vi "Ignore nearby.vi"(2 "Pixel messurments":dbl[][](array[numeric])=[[23.153969547670897, -111.544571524119, 21.215260576456764, -113.32770834490657, 24.840963307768085, -109.79999757930636, 5.058701764442134, 2.0870321222371477], [23.050654694780935, -101.06514097376787, 21.607228439301235, -101.66666442528367, 24.351003479212505, -100.29477690532804, 3.0676337521043995, 16.638621652215505], [26.166824298370553, -72.64693767062666, 25.428915102034793, -73.44497830048203, 26.800802621990428, -71.87710684910417, 2.0833377679713307, 56.22134914640533], [29.98722136986337, -92.77263364027391, 29.544577661901695, -94.41525896266103, 30.426505353301746, -91.67148392274976, 2.8820301737661103, 93.58353525070883], [33.497201865026476, -86.57562011966348, 31.3084330447018, -87.45782939717174, 35.424095604568706, -85.39999811723828, 4.6014506281565986, 14.316750347188261], [33.5765445343372, -116.26011097886011, 31.896384838968494, -116.95341107621789, 35.4240956045687, -115.67951552197337, 3.750673689999642, 171.9805540666988], [38.33864305074378, -21.110133273436578, 37.0899590216577, -22.881123993545778, 39.931726027280085, -19.353413227945573, 4.529942931205161, 120.31992372552097], [40.0072805802987, -113.89413853927944, 38.9518063701689, -114.79758783057333, 40.81365371868012, -112.73975655063988, 2.775093714783486, 47.83521789725366], [41.038596937087156, -58.27234689395295, 40.42168585583566, -59.922087032347925, 41.891565341502414, -56.00240840390325, 4.186218610234045, 73.82475304681395], [45.0319078671391, -81.3913267852408, 44.04738858714698, -82.4602391459048, 46.00722790136932, -80.20642393454911, 2.9867462470905948, 50.627358900913684], [48.95238800468319, -102.12113110093198, 48.261043112725, -103.43051980808379, 49.534938666969516, -100.68674476817252, 3.0250803878184858, 94.7160819713975], [51.907561130887736, -82.82818937012169, 51.20080208405851, -83.93011863157155, 52.572689604014144, -81.8722873516381, 2.4732053986845846, 57.35545946274767], [58.16901076576446, -83.11221235775318, 57.27630395814775, -84.51807042583825, 59.04015934094785, -81.67630342021586, 3.3446712133895797, 115.97608069015298], [59.765299887202126, -69.69094378329712, 58.060239683836684, -72.26907471194865, 61.685942415148006, -67.46746839210392, 6.016738613784976, 59.86524109532162], [59.34002546551593, -97.34457616713128, 58.158231649547794, -99.70682511106135, 60.90200668945907, -95.2971866540611, 5.1935741826891935, 122.23317974279698], [61.1549553545596, -135.6886543755193, 58.746183443814495, -137.72770780697465, 63.939757626503685, -133.3180693499744, 6.8130847721536005, 15.222386784548284], [59.62811113521553, -72.96668418213245, 58.942167375236735, -73.83694616332652, 60.31405489519237, -72.36706667765976, 2.0106270339856613, 48.415236976347224], [62.824559752547245, -84.35320972876715, 62.07791027799247, -85.3999981172383, 63.93975762650369, -83.44015880301596, 2.703228752201658, 55.070701538642446], [67.50979258154165, -35.983900770382576, 66.19357283785939, -36.893975090235486, 68.83935591205955, -34.93413577601315, 3.2925883759278944, 28.854486763895764], [70.58563258349632, -102.94916232772741, 70.11325146630405, -103.92047963663937, 70.9951791577041, -102.05863228812815, 2.0601631008287864, 90.85123906790069], [72.09966487288538, -135.68357879336168, 70.70120326057074, -136.45381225273013, 73.444978300482, -134.98393276706338, 3.112691306895698, 158.10400496188345], [74.93335976567708, -53.65471277783657, 73.73895419761537, -54.72851284965874, 76.09076137468217, -52.180721741169705, 3.4673096963782624, 79.81300563717497], [81.4765115108334, -135.9072404854036, 80.89236769452688, -137.2377479784191, 82.06827128306028, -134.68995686993006, 2.806062861380964, 84.7022174765496], [86.0399891231283, -50.73731834562851, 84.71405435726045, -51.78875387832524, 87.55582136288284, -49.63293063268067, 3.566961393217694, 34.49100372630609], [86.52149180204897, -127.56713202513569, 85.49799008294937, -128.32047909870747, 87.65381332859394, -126.75260764732958, 2.665669663425548, 142.89159787285385], [87.31640917394765, -95.77322716932507, 86.37991777434944, -96.66907417401673, 88.14377315714954, -94.61124289408328, 2.7103238529934846, 57.3397049555742], [90.69523063175343, -49.389283942453375, 89.90762853994964, -50.80883422121407, 91.47549999132751, -48.0650591813028, 3.1601459393018283, 67.85295326199508], [91.47767759056437, -38.45930600916872, 90.59357229992747, -39.83373406156899, 92.25943571701644, -37.38393491879107, 2.9625355296351765, 67.4436053938025], [91.6756439590325, -110.08519117762921, 90.98554016277193, -111.46586099639536, 92.35742768272756, -108.82007792219521, 2.9803092864892458, 73.2743292894458], [94.97610203064093, -79.2583337845439, 93.92529913410543, -81.38232752308251, 96.08112237975, -77.2666649632156, 4.646100749354419, 82.72828659799865], [95.55597452715126, -53.02657057247167, 94.41525896266101, -53.84658515825869, 96.76706613972782, -52.27871370688082, 2.826520455639525, 27.994921080233407], [97.52458601055257, -59.89827657686741, 95.98313041403888, -61.48995848372581, 99.0208813510835, -58.06023968383672, 4.58158289260689, 67.83670357667657], [104.04356927261908, -97.09280280543281, 102.15662425383924, -99.31485724821688, 106.37027877941726, -95.2971866540611, 5.82207535712724, 139.97342300498846], [105.6341245242916, -56.8165471327239, 103.43051980808376, -59.62811113521459, 107.44819040223955, -54.14056105539205, 6.8010942414955915, 97.24255309011542], [108.74034645194116, -27.947236302017327, 107.15421450510621, -29.05461783334615, 110.09397347643971, -26.800802621990464, 3.7043036884783214, 179.48800650814684], [108.94516822485872, -101.74905431831091, 107.44819040223955, -103.03855194523932, 110.38794937357305, -100.29477690532805, 4.021254067971323, 134.86479080046723], [108.19190180442153, -38.31485859305124, 107.54618236795066, -40.4216858558357, 108.8200779221952, -36.40401526167991, 4.214793813019577, 95.766849041926], [113.34632336244485, -120.71810593844376, 108.33011809363958, -129.1044148243964, 119.99116201326248, -113.03373244777325, 19.855648499751403, 117.93513609604776], [110.89988870847331, -36.10088123691543, 110.19196544215083, -37.38393491879108, 111.95582082495093, -34.93413577601316, 3.01872516990009, 118.34762931907156], [112.12384659651235, -141.66925469877293, 110.1919654421508, -142.5293141268194, 113.81766817346212, -140.66746677830818, 4.075806158908521, 154.94585244328283], [111.94393422553061, -111.33684790541606, 111.17188509926198, -112.64176458492877, 112.93574048206209, -109.8979895450175, 3.261822693077137, 80.35839913755879], [113.17320881710795, -56.74212824263561, 112.05381279066204, -57.76626378670337, 114.50361193343996, -55.806424472481034, 3.1372736535927026, 35.50013253075657], [113.35459839606153, -104.14071410499425, 112.24979672208427, -105.39035912230612, 114.69959586486219, -103.23453587666155, 3.263294302758627, 143.00507300986496], [113.19783010478292, -99.25886183936566, 112.54377261921762, -100.0008010081947, 114.11164407059549, -98.53092152252795, 2.149131589835694, 47.55595083581141], [116.66657407075296, -129.615181166239, 114.69959586486218, -131.84818986430767, 118.9132503904402, -127.83051927015187, 5.8220753571272486, 34.29865811759245], [117.22479297101977, -102.7280748104678, 116.65943517908453, -104.21445553377274, 117.73734680190681, -100.78473673388365, 3.5951167592900255, 99.12601563426801], [117.88310678098033, -27.52604140581268, 116.85541911050677, -30.034537490457318, 119.01124235615134, -24.351003479212544, 6.078662083340181, 88.17913237932774], [120.27203997437059, -29.277282745526623, 119.59919415041804, -30.132529456168434, 121.0690736360848, -28.564658004790566, 2.149131589835694, 134.80702391388525], [122.37824080821565, -66.95925515815723, 120.77509773895143, -67.76144428923729, 123.81284867599605, -66.0955808721483, 3.4645391728065165, 2.419559816356106], [124.22781044838646, -130.0453519753959, 120.97108167037365, -133.41606131568554, 127.14457551017401, -126.94859157875183, 8.940927859467736, 49.997547132224106], [127.11854733497613, -75.26923831502631, 121.46104149892925, -85.79196598008278, 133.02409345284104, -64.9196772836149, 23.861194561831226, 100.51933634071696], [123.44513135008438, -88.742489220347, 121.55903346464036, -90.49558033421638, 125.08674423024057, -86.67389367148283, 5.200964544567394, 127.6966770746937], [123.85620676494109, -112.66471886731529, 122.83292901888488, -114.11164407059553, 124.79276833310722, -111.26987706497314, 3.452044300384267, 90.633155429399], [124.9514844539646, -25.088566629005186, 123.81284867599607, -26.89879458770158, 126.06666388735175, -23.371083822101376, 4.186218610234045, 93.52218227931537], [125.59434261258917, -97.05761231803307, 124.59678440168499, -98.04096169397238, 126.4586317501962, -96.17911434546116, 2.6330497713329524, 129.10781173086656], [127.40158171115596, -115.12378229825315, 126.06666388735174, -116.8554191105068, 128.9084308929741, -113.22971637919548, 4.606664738189911, 58.13558778744161], [128.23124963877498, -34.471450789306296, 127.24256747588515, -35.914055433124325, 129.10441482439637, -33.07228842750194, 3.397368873614151, 107.02312092204234], [129.10060076613485, -65.4422033045112, 128.32047909870744, -66.29156480357054, 129.8883505500853, -64.72369335219267, 2.2173050705961703, 39.82366841561815], [133.78792767072648, -31.77990687124756, 130.08433448150754, -35.13011970743539, 137.04176404699683, -29.15260979905727, 9.17259237421478, 123.5919624202362], [133.52789338380413, -130.03809978431872, 130.86827020719645, -133.2200773842633, 136.355820287019, -126.85059961304071, 8.407345178869432, 105.15474563599331], [133.4386543999588, -76.84519319023414, 132.24015772715208, -79.61847214028242, 134.4939729385078, -74.32690599188211, 5.75155242607024, 105.42860515334493], [136.10731294416433, -56.13063043246762, 133.71003721281886, -59.628111135214596, 138.80561942979693, -53.65060122683647, 7.854653578277136, 114.24744088018468], [138.67403021873304, -30.05693565405594, 138.11967566981912, -31.210441078990723, 139.1975872926414, -28.956625867635037, 2.498314726681498, 111.14098598849264]], 3 "Raw par mes.":dbl[][](array[numeric])=[[23.153969547670897, -111.544571524119, 21.215260576456764, -113.32770834490657, 24.840963307768085, -109.79999757930636, 5.058701764442134, 2.0870321222371477], [23.050654694780935, -101.06514097376787, 21.607228439301235, -101.66666442528367, 24.351003479212505, -100.29477690532804, 3.0676337521043995, 16.638621652215505], [26.166824298370553, -72.64693767062666, 25.428915102034793, -73.44497830048203, 26.800802621990428, -71.87710684910417, 2.0833377679713307, 56.22134914640533], [29.98722136986337, -92.77263364027391, 29.544577661901695, -94.41525896266103, 30.426505353301746, -91.67148392274976, 2.8820301737661103, 93.58353525070883], [33.497201865026476, -86.57562011966348, 31.3084330447018, -87.45782939717174, 35.424095604568706, -85.39999811723828, 4.6014506281565986, 14.316750347188261], [33.5765445343372, -116.26011097886011, 31.896384838968494, -116.95341107621789, 35.4240956045687, -115.67951552197337, 3.750673689999642, 171.9805540666988], [38.33864305074378, -21.110133273436578, 37.0899590216577, -22.881123993545778, 39.931726027280085, -19.353413227945573, 4.529942931205161, 120.31992372552097], [40.0072805802987, -113.89413853927944, 38.9518063701689, -114.79758783057333, 40.81365371868012, -112.73975655063988, 2.775093714783486, 47.83521789725366], [41.038596937087156, -58.27234689395295, 40.42168585583566, -59.922087032347925, 41.891565341502414, -56.00240840390325, 4.186218610234045, 73.82475304681395], [45.0319078671391, -81.3913267852408, 44.04738858714698, -82.4602391459048, 46.00722790136932, -80.20642393454911, 2.9867462470905948, 50.627358900913684], [48.95238800468319, -102.12113110093198, 48.261043112725, -103.43051980808379, 49.534938666969516, -100.68674476817252, 3.0250803878184858, 94.7160819713975], [51.907561130887736, -82.82818937012169, 51.20080208405851, -83.93011863157155, 52.572689604014144, -81.8722873516381, 2.4732053986845846, 57.35545946274767], [58.16901076576446, -83.11221235775318, 57.27630395814775, -84.51807042583825, 59.04015934094785, -81.67630342021586, 3.3446712133895797, 115.97608069015298], [59.765299887202126, -69.69094378329712, 58.060239683836684, -72.26907471194865, 61.685942415148006, -67.46746839210392, 6.016738613784976, 59.86524109532162], [59.34002546551593, -97.34457616713128, 58.158231649547794, -99.70682511106135, 60.90200668945907, -95.2971866540611, 5.1935741826891935, 122.23317974279698], [61.1549553545596, -135.6886543755193, 58.746183443814495, -137.72770780697465, 63.939757626503685, -133.3180693499744, 6.8130847721536005, 15.222386784548284], [59.62811113521553, -72.96668418213245, 58.942167375236735, -73.83694616332652, 60.31405489519237, -72.36706667765976, 2.0106270339856613, 48.415236976347224], [62.824559752547245, -84.35320972876715, 62.07791027799247, -85.3999981172383, 63.93975762650369, -83.44015880301596, 2.703228752201658, 55.070701538642446], [67.50979258154165, -35.983900770382576, 66.19357283785939, -36.893975090235486, 68.83935591205955, -34.93413577601315, 3.2925883759278944, 28.854486763895764], [70.58563258349632, -102.94916232772741, 70.11325146630405, -103.92047963663937, 70.9951791577041, -102.05863228812815, 2.0601631008287864, 90.85123906790069], [72.09966487288538, -135.68357879336168, 70.70120326057074, -136.45381225273013, 73.444978300482, -134.98393276706338, 3.112691306895698, 158.10400496188345], [74.93335976567708, -53.65471277783657, 73.73895419761537, -54.72851284965874, 76.09076137468217, -52.180721741169705, 3.4673096963782624, 79.81300563717497], [81.4765115108334, -135.9072404854036, 80.89236769452688, -137.2377479784191, 82.06827128306028, -134.68995686993006, 2.806062861380964, 84.7022174765496], [86.0399891231283, -50.73731834562851, 84.71405435726045, -51.78875387832524, 87.55582136288284, -49.63293063268067, 3.566961393217694, 34.49100372630609], [86.52149180204897, -127.56713202513569, 85.49799008294937, -128.32047909870747, 87.65381332859394, -126.75260764732958, 2.665669663425548, 142.89159787285385], [87.31640917394765, -95.77322716932507, 86.37991777434944, -96.66907417401673, 88.14377315714954, -94.61124289408328, 2.7103238529934846, 57.3397049555742], [90.69523063175343, -49.389283942453375, 89.90762853994964, -50.80883422121407, 91.47549999132751, -48.0650591813028, 3.1601459393018283, 67.85295326199508], [91.47767759056437, -38.45930600916872, 90.59357229992747, -39.83373406156899, 92.25943571701644, -37.38393491879107, 2.9625355296351765, 67.4436053938025], [91.6756439590325, -110.08519117762921, 90.98554016277193, -111.46586099639536, 92.35742768272756, -108.82007792219521, 2.9803092864892458, 73.2743292894458], [94.97610203064093, -79.2583337845439, 93.92529913410543, -81.38232752308251, 96.08112237975, -77.2666649632156, 4.646100749354419, 82.72828659799865], [95.55597452715126, -53.02657057247167, 94.41525896266101, -53.84658515825869, 96.76706613972782, -52.27871370688082, 2.826520455639525, 27.994921080233407], [97.52458601055257, -59.89827657686741, 95.98313041403888, -61.48995848372581, 99.0208813510835, -58.06023968383672, 4.58158289260689, 67.83670357667657], [104.04356927261908, -97.09280280543281, 102.15662425383924, -99.31485724821688, 106.37027877941726, -95.2971866540611, 5.82207535712724, 139.97342300498846], [105.6341245242916, -56.8165471327239, 103.43051980808376, -59.62811113521459, 107.44819040223955, -54.14056105539205, 6.8010942414955915, 97.24255309011542], [108.74034645194116, -27.947236302017327, 107.15421450510621, -29.05461783334615, 110.09397347643971, -26.800802621990464, 3.7043036884783214, 179.48800650814684], [108.94516822485872, -101.74905431831091, 107.44819040223955, -103.03855194523932, 110.38794937357305, -100.29477690532805, 4.021254067971323, 134.86479080046723], [108.19190180442153, -38.31485859305124, 107.54618236795066, -40.4216858558357, 108.8200779221952, -36.40401526167991, 4.214793813019577, 95.766849041926], [113.34632336244485, -120.71810593844376, 108.33011809363958, -129.1044148243964, 119.99116201326248, -113.03373244777325, 19.855648499751403, 117.93513609604776], [110.89988870847331, -36.10088123691543, 110.19196544215083, -37.38393491879108, 111.95582082495093, -34.93413577601316, 3.01872516990009, 118.34762931907156], [112.12384659651235, -141.66925469877293, 110.1919654421508, -142.5293141268194, 113.81766817346212, -140.66746677830818, 4.075806158908521, 154.94585244328283], [111.94393422553061, -111.33684790541606, 111.17188509926198, -112.64176458492877, 112.93574048206209, -109.8979895450175, 3.261822693077137, 80.35839913755879], [113.17320881710795, -56.74212824263561, 112.05381279066204, -57.76626378670337, 114.50361193343996, -55.806424472481034, 3.1372736535927026, 35.50013253075657], [113.35459839606153, -104.14071410499425, 112.24979672208427, -105.39035912230612, 114.69959586486219, -103.23453587666155, 3.263294302758627, 143.00507300986496], [113.19783010478292, -99.25886183936566, 112.54377261921762, -100.0008010081947, 114.11164407059549, -98.53092152252795, 2.149131589835694, 47.55595083581141], [116.66657407075296, -129.615181166239, 114.69959586486218, -131.84818986430767, 118.9132503904402, -127.83051927015187, 5.8220753571272486, 34.29865811759245], [117.22479297101977, -102.7280748104678, 116.65943517908453, -104.21445553377274, 117.73734680190681, -100.78473673388365, 3.5951167592900255, 99.12601563426801], [117.88310678098033, -27.52604140581268, 116.85541911050677, -30.034537490457318, 119.01124235615134, -24.351003479212544, 6.078662083340181, 88.17913237932774], [120.27203997437059, -29.277282745526623, 119.59919415041804, -30.132529456168434, 121.0690736360848, -28.564658004790566, 2.149131589835694, 134.80702391388525], [122.37824080821565, -66.95925515815723, 120.77509773895143, -67.76144428923729, 123.81284867599605, -66.0955808721483, 3.4645391728065165, 2.419559816356106], [124.22781044838646, -130.0453519753959, 120.97108167037365, -133.41606131568554, 127.14457551017401, -126.94859157875183, 8.940927859467736, 49.997547132224106], [127.11854733497613, -75.26923831502631, 121.46104149892925, -85.79196598008278, 133.02409345284104, -64.9196772836149, 23.861194561831226, 100.51933634071696], [123.44513135008438, -88.742489220347, 121.55903346464036, -90.49558033421638, 125.08674423024057, -86.67389367148283, 5.200964544567394, 127.6966770746937], [123.85620676494109, -112.66471886731529, 122.83292901888488, -114.11164407059553, 124.79276833310722, -111.26987706497314, 3.452044300384267, 90.633155429399], [124.9514844539646, -25.088566629005186, 123.81284867599607, -26.89879458770158, 126.06666388735175, -23.371083822101376, 4.186218610234045, 93.52218227931537], [125.59434261258917, -97.05761231803307, 124.59678440168499, -98.04096169397238, 126.4586317501962, -96.17911434546116, 2.6330497713329524, 129.10781173086656], [127.40158171115596, -115.12378229825315, 126.06666388735174, -116.8554191105068, 128.9084308929741, -113.22971637919548, 4.606664738189911, 58.13558778744161], [128.23124963877498, -34.471450789306296, 127.24256747588515, -35.914055433124325, 129.10441482439637, -33.07228842750194, 3.397368873614151, 107.02312092204234], [129.10060076613485, -65.4422033045112, 128.32047909870744, -66.29156480357054, 129.8883505500853, -64.72369335219267, 2.2173050705961703, 39.82366841561815], [133.78792767072648, -31.77990687124756, 130.08433448150754, -35.13011970743539, 137.04176404699683, -29.15260979905727, 9.17259237421478, 123.5919624202362], [133.52789338380413, -130.03809978431872, 130.86827020719645, -133.2200773842633, 136.355820287019, -126.85059961304071, 8.407345178869432, 105.15474563599331], [133.4386543999588, -76.84519319023414, 132.24015772715208, -79.61847214028242, 134.4939729385078, -74.32690599188211, 5.75155242607024, 105.42860515334493], [136.10731294416433, -56.13063043246762, 133.71003721281886, -59.628111135214596, 138.80561942979693, -53.65060122683647, 7.854653578277136, 114.24744088018468], [138.67403021873304, -30.05693565405594, 138.11967566981912, -31.210441078990723, 139.1975872926414, -28.956625867635037, 2.498314726681498, 111.14098598849264]]) -> (0 "Picking array":dbl[][](array[numeric]), 1 "Sorted data array":dbl[][](array[numeric]))   [LabVIEW 2024]
doc: "This Vi removes from object array if they are closer together than 5mm"
uses:
  1cb59190-bcf4-462b-bc26-c9ba3c9ce25d.vi
  <vilib>/Array/Sort 2D Array - Pop Stack.vi
  <vilib>/Array/Sort 2D Array - Push Stack.vi
  1cb59190-bcf4-462b-bc26-c9ba3c9ce25d.vi/269d4b3b-47f5-49e3-8884-44851e4dd9d5.vi
  1cb59190-bcf4-462b-bc26-c9ba3c9ce25d.vi/6d99389c-673d-4efb-bf33-19b32bcf4cf8.vi
panel:
  out "Numeric":i32
  out "Array":bool[][](array[boolean])
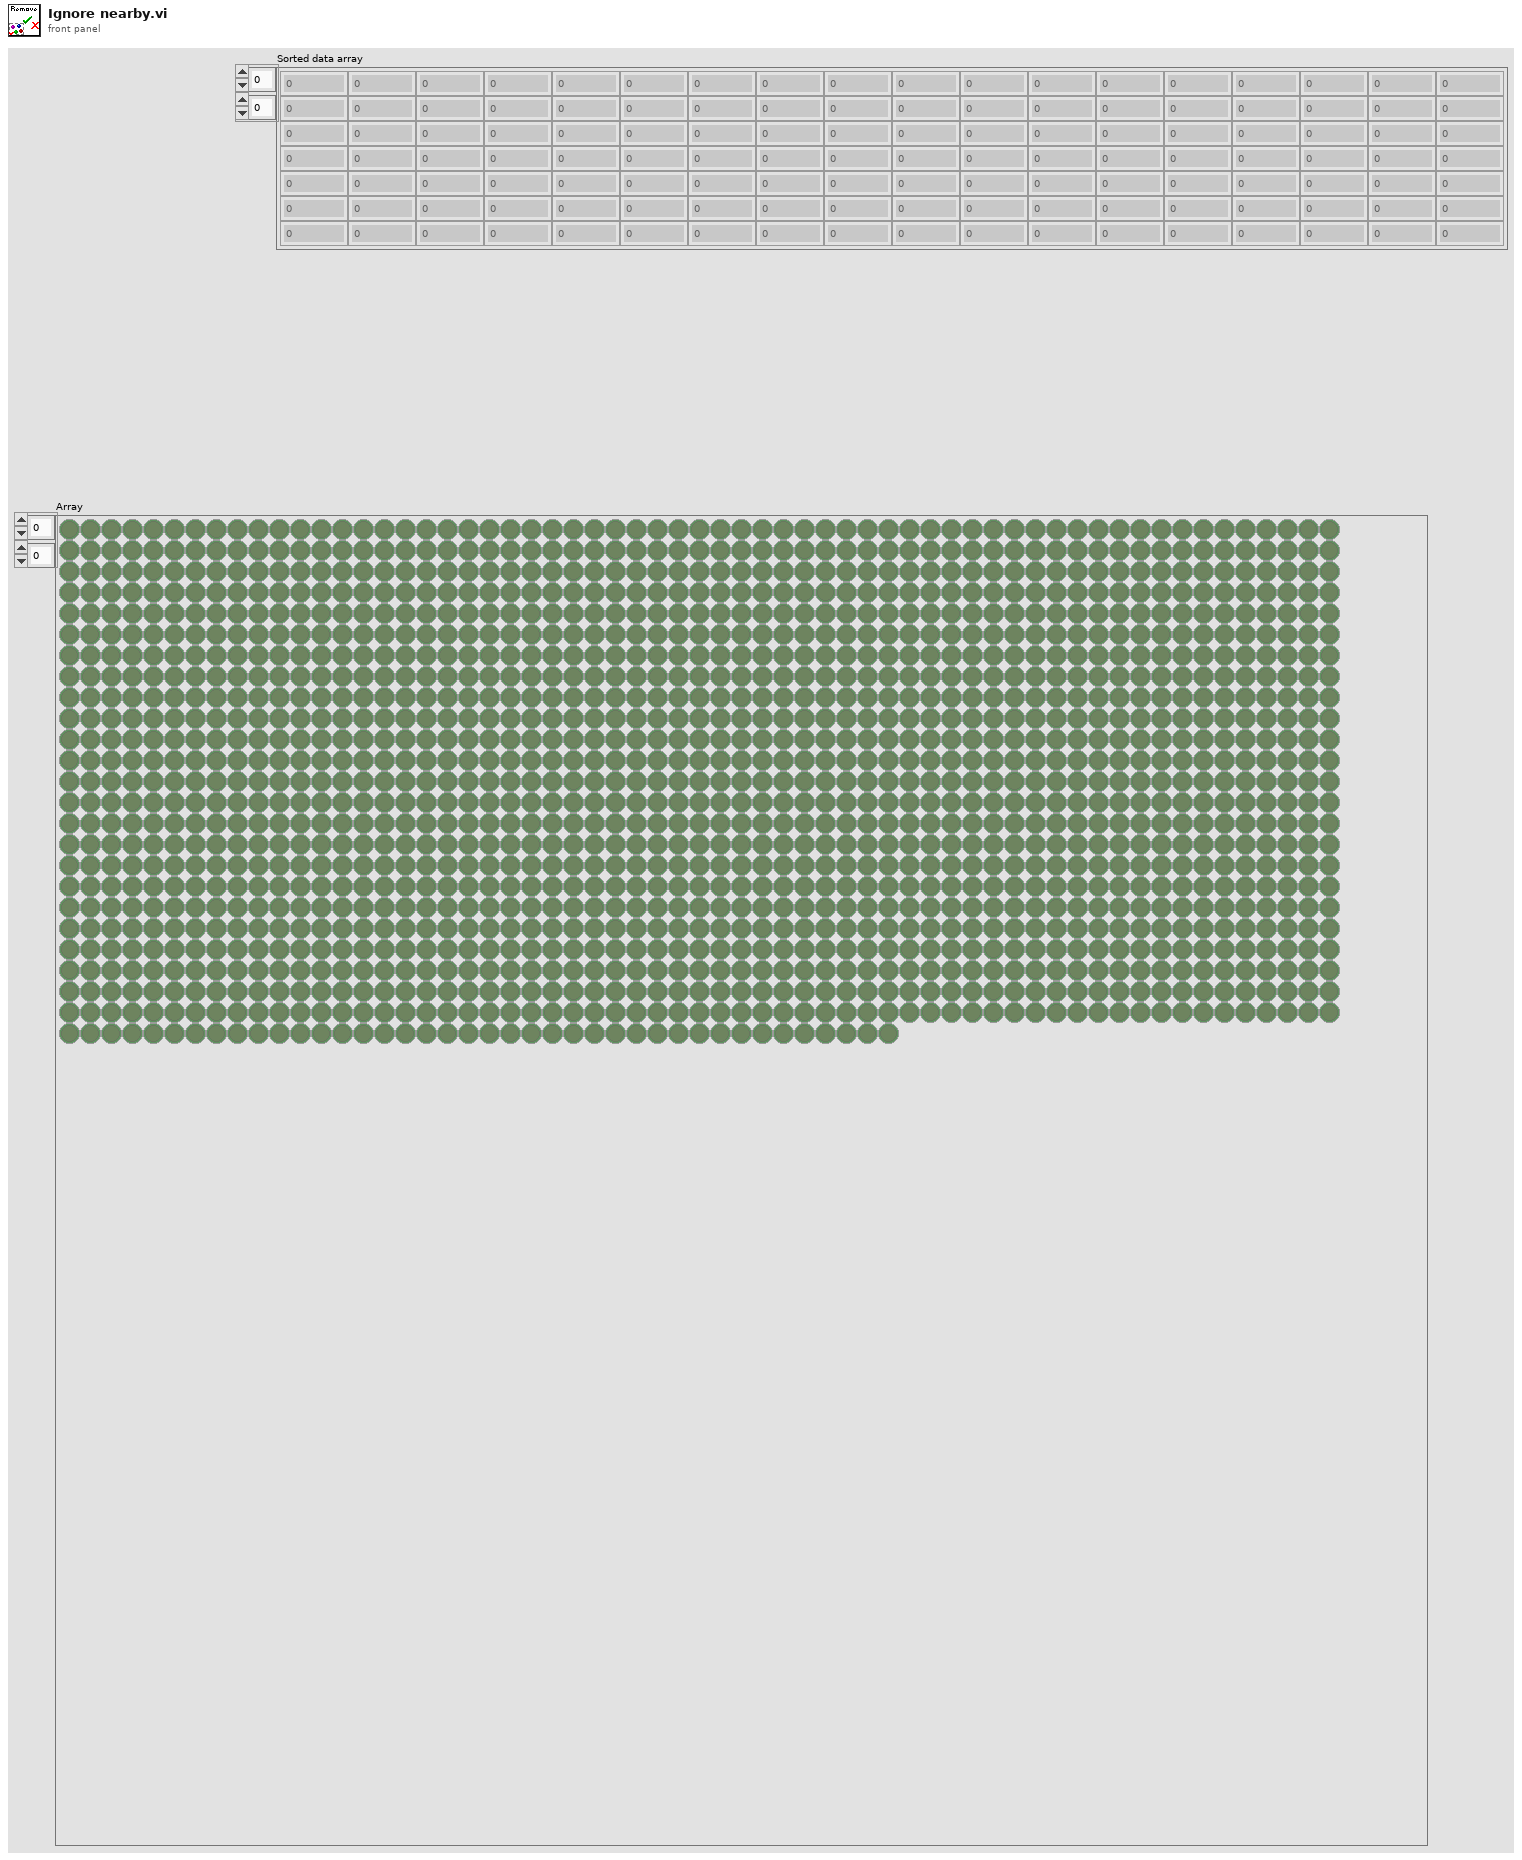
[diagram p1: front panel]
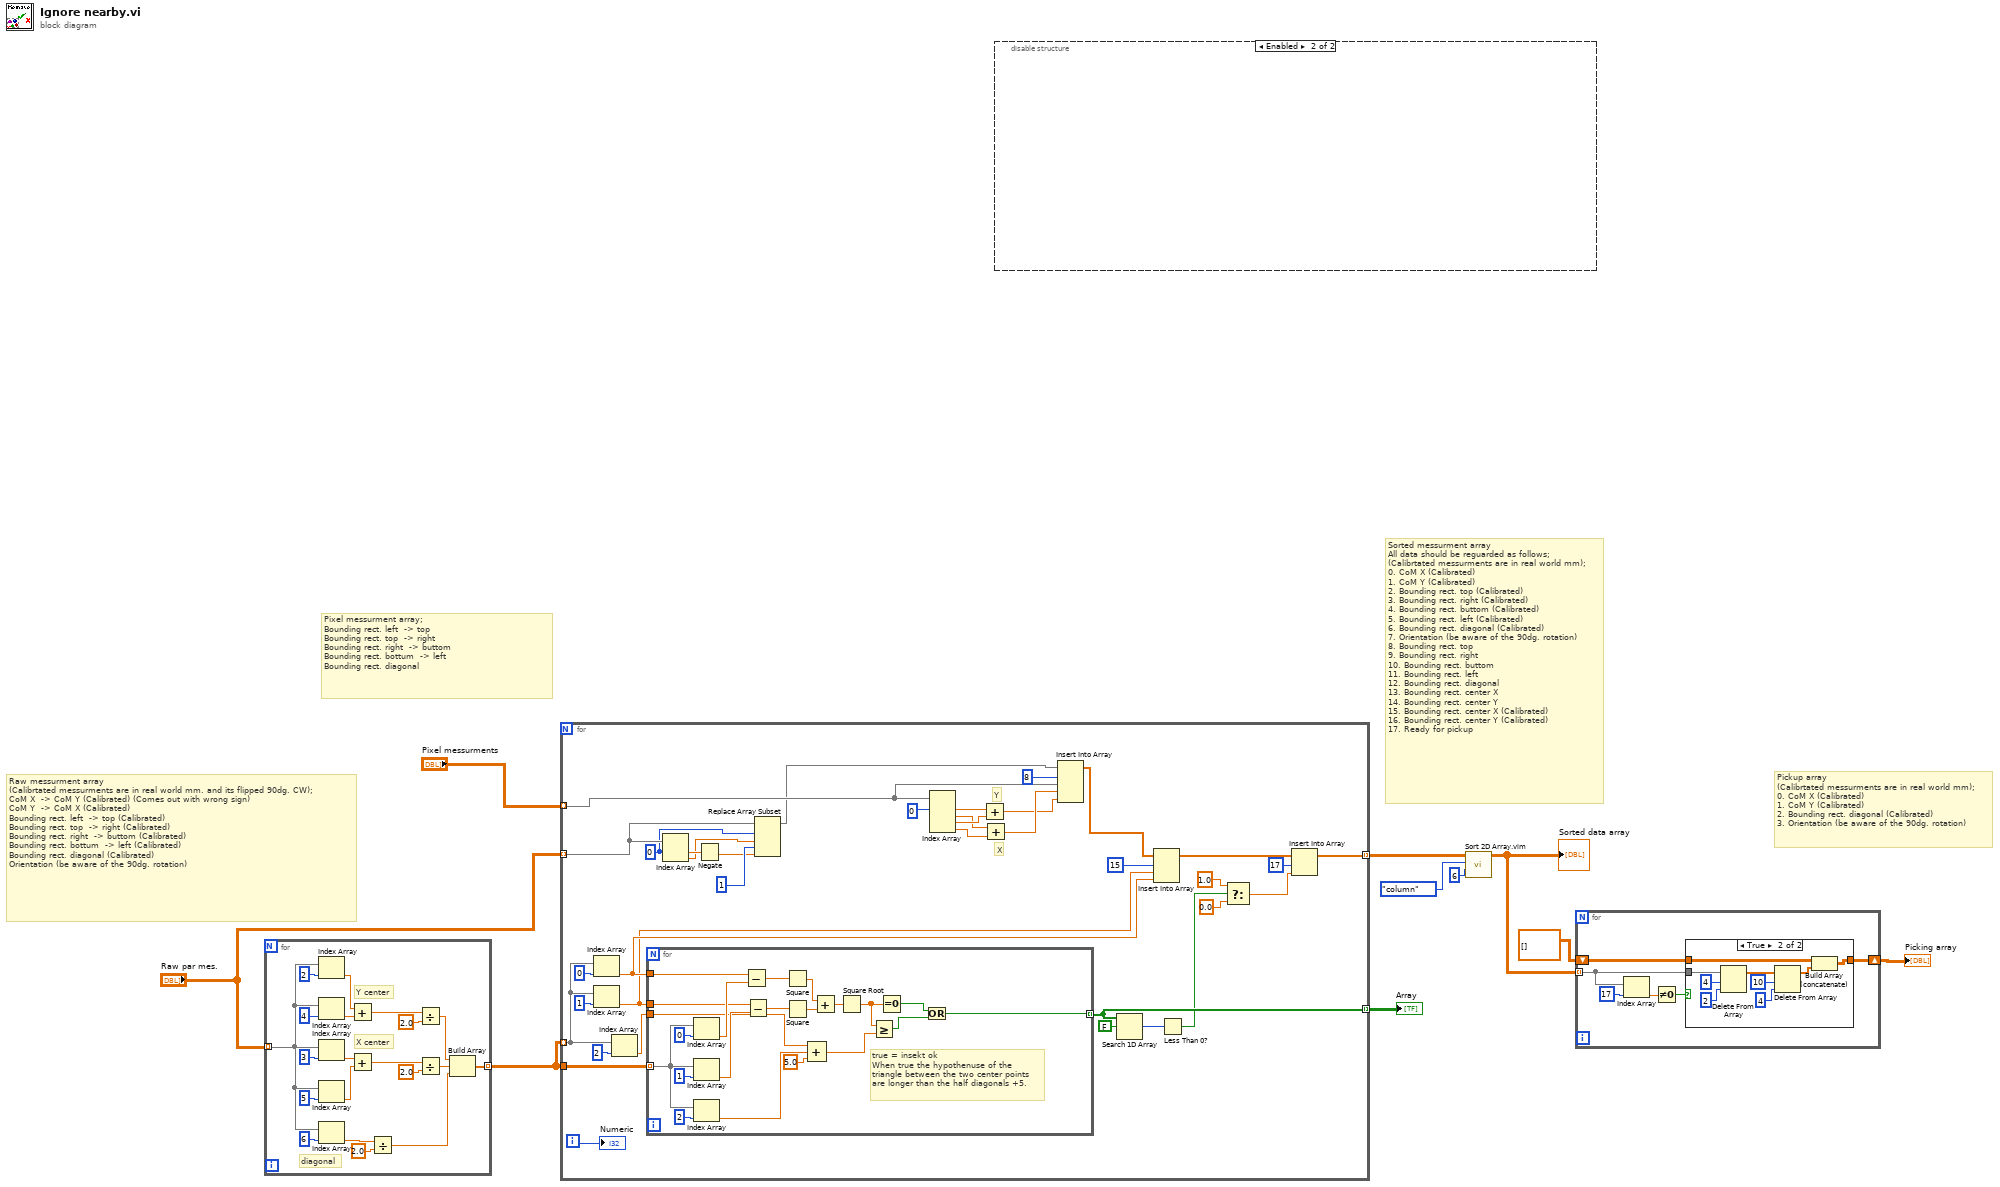
[diagram p0: block diagram]
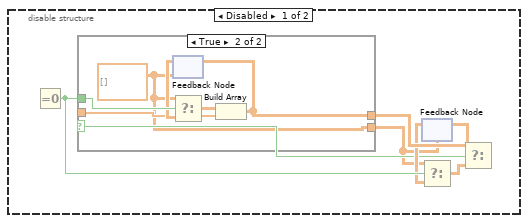
[diagram p3: hidden frame]
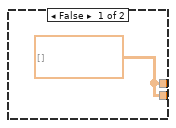
[diagram p4: hidden frame]
diagram:
  # "Pixel messurment array;\nBounding rect. left  -> top\nBounding rect. top  -> right\nBounding rect. right  -> buttom\nBounding rect. bottum  -> left\nBounding rect. diagonal"
  # "Pickup array\n(Calibrtated messurments are in real world mm);\n0. CoM X (Calibrated)\n1. CoM Y (Calibrated)\n2. Bounding rect. diagonal (Calibrated)\n3. Orientation (be aware of the 90dg. rotation)"
  # "Raw messurment array\n(Calibrtated messurments are in real world mm. and its flipped 90dg. CW);\nCoM X  -> CoM Y (Calibrated) (Comes out with wrong sign)\nCoM Y  -> CoM X (Calibrated)\nBounding rect. left  -> top (Calibrated)\nBounding rect. top  -> right (Calibrated)\nBounding rect. right  -> buttom (Calibrated)\nBounding rect. bottum  -> left (Calibrated)\nBounding rect. diagonal (Calibrated)\nOrientation (be aware of the 90dg. rotation)"
  # "Sorted messurment array\nAll data should be reguarded as follows;\n(Calibrtated messurments are in real world mm);\n0. CoM X (Calibrated)\n1. CoM Y (Calibrated)\n2. Bounding rect. top (Calibrated)\n3. Bounding rect. right (Calibrated)\n4. Bounding rect. buttom (Calibrated)\n5. Bounding rect. left (Calibrated)\n6. Bounding rect. diagonal (Calibrated)\n7. Orientation (be aware of the 90dg. rotation)\n8. Bounding rect. top\n9. Bounding rect. right\n10. Bounding rect. buttom\n11. Bounding rect. left\n12. Bounding rect. diagonal\n13. Bounding rect. center X\n14. Bounding rect. center Y\n15. Bounding rect. center X (Calibrated)\n16. Bounding rect. center Y (Calibrated)\n17. Ready for pickup"
  n1 = for {
    tunnel: "Raw par mes." -> [w17] mode=indexing
    tunnel: [w15] -> w10 mode=indexing
    # "diagonal"
    # "X center"
    # "Y center"
    n2 = Index Array(array=w17, index=2 ("index (row)")) -> (element=w25:dbl)
    n3 = Index Array(array=w17, index=4 ("index (row)")) -> (element=w28:dbl)
    n4 = Index Array(array=w17, index=3 ("index (row)")) -> (element=w24:dbl)
    n5 = Index Array(array=w17, index=5 ("index (row)")) -> (element=w21:dbl)
    n6 = Index Array(array=w17, index=6 ("index (row)")) -> (element=w12:dbl)
    n7 = Add(x=w25, y=w28) -> (x+y=w27:dbl)
    n8 = Add(x=w24, y=w21) -> (x+y=w22:dbl)
    n9 = Divide(x=w12, y=2.0) -> (x/y=w11:dbl)
    n10 = Divide(x=w27, y=2.0) -> (x/y=w16:dbl)
    n11 = Divide(x=w22, y=2.0) -> (x/y=w14:dbl)
    n12 = Build Array(w16, w14, w11) -> (w15:dbl[])
  }
  n13 = for {
    tunnel: w10 -> [w61] mode=indexing
    tunnel: w10 -> [w49]
    tunnel: "Raw par mes." -> [w36] mode=indexing
    tunnel: [w58] -> w5 mode=indexing
    tunnel: [w52] -> w8 mode=indexing
    tunnel: "Pixel messurments" -> [w41] mode=indexing
    i -> [w46]
    w34 = 0 ("index")
    # "X"
    # "Y"
    n14 = Index Array(array=w61, index=0 ("index (row)")) -> (element=w54:dbl)
    n15 = Index Array(array=w61, index=1 ("index (row)")) -> (element=w53:dbl)
    n16 = Index Array(array=w61, index=2) -> (element=w64:dbl)
    n17 = for {
      tunnel: w49 -> [w85] mode=indexing
      tunnel: w54 -> [w84]
      tunnel: w53 -> [w81]
      tunnel: w64 -> [w75]
      tunnel: [w68] -> w52 mode=indexing
      # "true = insekt ok\nWhen true the hypothenuse of the\ntriangle between the two center points\nare longer than the half diagonals +5."
      n18 = Index Array(array=w85, index=0 ("index (row)")) -> (element=w83:dbl)
      n19 = Index Array(array=w85, index=1 ("index (row)")) -> (element=w80:dbl)
      n20 = Index Array(array=w85, index=2) -> (element=w74:dbl)
      n21 = Subtract(x=w84, y=w83) -> (x-y=w82:dbl)
      n22 = Subtract(x=w81, y=w80) -> (x-y=w79:dbl)
      n23 = Square(x=w82) -> (x^2=w78:dbl)
      n24 = Square(x=w79) -> (x^2=w77:dbl)
      n25 = Compound Arithmetic op=ADD(w75, w74, 5.0 ("value")) -> (w72:dbl)
      n26 = Add(x=w78, y=w77) -> (x+y=w76:dbl)
      n27 = Square Root(x=w76) -> (sqrt(x)=w69:dbl)
      n28 = Greater Or Equal?(x=w69, y=w72) -> (x >= y?=w71:bool)
      n29 = Equal To 0?(x=w69) -> (x = 0?=w70:bool)
      n30 = Or(x=w70, y=w71) -> (x .or. y?=w68:bool)
    }
    n31 = Index Array(array=w36, index #1=w34) -> (element #1=w37:dbl, element #2=w31:dbl)  [unwired: 1 in]
    n32 = Negate(x=w37) -> (-x=w32:dbl)
    n33 = Replace Array Subset(array=w36, new element #1=w31, index #1=w34, new element #2=w32, index #2=1) -> (w35:dbl[])
    n34 = Index Array(array=w41, index #1=0 ("index")) -> (element #1=w45:dbl, element #2=w43:dbl, element #3=w44:dbl, element #4=w42:dbl)  [unwired: 3 in]
    n35 = Add(x=w45, y=w44) -> (x+y=w39:dbl)
    n36 = Add(x=w43, y=w42) -> (x+y=w40:dbl)
    n37 = Insert Into Array(array=w35, index=8, new element #1=w41, new element #2=w40, new element #3=w39) -> (w38:dbl[])
    n38 = Search 1D Array(1D array=w52, element=FALSE) -> (index of element=w51:i32)  [unwired: 1 in]
    n39 = Insert Into Array(array=w38, index=15, new element #1=w53, new element #2=w54) -> (w60:dbl[])
    n40 = Less Than 0?(x=w51) -> (x < 0?=w50:bool)
    n41 = Select(t=1.0, s=w50, f=0.0) -> (s? t:f=w59:dbl)
    n42 = Insert Into Array(array=w60, index=17, new element=w59) -> (w58:dbl[])
    "Numeric" <- w46
  }
  "Array" <- w8
  n43 = disable-structure shown="Enabled" {
    frame Disabled {
      n44 = Equal To 0?() -> (x = 0?=w94:bool)  [unwired: 1 in]
      n45 = case shown="True" w90 {
        tunnel: w94 -> [_ w102]
        tunnel: _ -> [_ w99]
        tunnel: [w96 w98] -> w95
        tunnel: [w96 w97] -> w89
        frame False {
          w96 = dbl[][] []
        }
        frame True {
          w97 = dbl[][] []
          n46 = feedback #1(w97) -> (w100:dbl[][])
          n47 = Select(t=w97, s=w102, f=w100) -> (s? t:f=w101:dbl[][])
          n48 = Build Array(w101, w99) -> (w98:dbl[][][])
          n49 = feedback-in #1(w98) -> ()
        }
      }
      n50 = feedback #2(w89) -> (w93:dbl[][])
      n51 = Select(t=w89, s=w94, f=w93) -> (s? t:f=w92:dbl[][])
      n52 = Select(t=w95, f=w92) -> (s=w90:bool, s? t:f=w91:dbl[][][])
      n53 = feedback-in #2(w91) -> ()
    }
    frame Enabled {
    }
  }
  n54 = call "Sort 2D Array.vim"("index"=6, "dimension to index (column)"=enum16{"column", "row"}."column", "2D array"=w5) -> ("sorted 2D array"=w4:dbl[][])  [unwired: 7 in, 1 out]
  "Sorted data array" <- w4
  n55 = for {
    tunnel: w4 -> [w105] mode=indexing
    shift-right: [w103] -> w2
    shift-left: dbl[][] [] -> [w104]
    n56 = Index Array(array=w105, index=17) -> (element=w107:dbl)
    n57 = Not Equal To 0?(x=w107) -> (x != 0?=w106:bool)
    n58 = case shown="True" w106 {
      tunnel: w105 -> [_ w116]
      tunnel: [w109 w118] -> w103
      tunnel: w104 -> [w109 w117]
      frame False {
      }
      frame True {
        n59 = Delete From Array(array=w116, length=4 ("index"), index=2) -> (array with subset deleted=w111:dbl[])  [unwired: 1 out]
        n60 = Delete From Array(array=w111, length=10 ("index"), index=4) -> (array with subset deleted=w110:dbl[])  [unwired: 1 out]
        n61 = Build Array (concatenate)(w117, w110) -> (w118:dbl[][])
      }
    }
  }
  "Picking array" <- w2
